vi "VISJS Viewer.vi"(4 "Extra Scripts":string, 5 "FileDependency In":map{path, T1}(c390), 6 "Options":string, 7 "OpenWebBrowser(False)":bool, 8 "error in":errorcluster, 9 "Embedd VISJS Librarya in HTMl File(False)":bool, 10 "HTMLFilePath":path, 11 "LibraryDependency":map{path, T3}(c390)) -> (0 "error out":errorcluster, 3 "HTMLFileContent":string)   [LabVIEW 2020, in "VISJS Viewer.lvlib"] (continued)
{key:\"_setPixelRatio\",value:function(){this.pixelRatio=this._determinePixelRatio()}},{key:\"setTransform\",value:function(){var g=this.getContext();if(void 0===g)throw new Error(\"Could not get canvax context\");g.setTransform(this.pixelRatio,0,0,this.pixelRatio,0,0)}},{key:\"_XconvertDOMtoCanvas\",value:function(g){return(g-this.body.view.translation.x)/this.body.view.scale}},{key:\"_XconvertCanvasToDOM\",value:function(g){return g*this.body.view.scale+this.body.view.translation.x}},{key:\"_YconvertDOMtoCanvas\",value:function(g){return(g-this.body.view.translation.y)/this.body.view.scale}},{key:\"_YconvertCanvasToDOM\",value:function(g){return g*this.body.view.scale+this.body.view.translation.y}},{key:\"canvasToDOM\",value:function(g){return{x:this._XconvertCanvasToDOM(g.x),y:this._YconvertCanvasToDOM(g.y)}}},{key:\"DOMtoCanvas\",value:function(g){return{x:this._XconvertDOMtoCanvas(g.x),y:this._YconvertDOMtoCanvas(g.y)}}}]),g}();var IP=function(){function g(t,A){var e,C,I=this;cn(this,g),this.body=t,this.canvas=A,this.animationSpeed=1/this.renderRefreshRate,this.animationEasingFunction=\"easeInOutQuint\",this.easingTime=0,this.sourceScale=0,this.targetScale=0,this.sourceTranslation=0,this.targetTranslation=0,this.lockedOnNodeId=void 0,this.lockedOnNodeOffset=void 0,this.touchTime=0,this.viewFunction=void 0,this.body.emitter.on(\"fit\",je(e=this.fit).call(e,this)),this.body.emitter.on(\"animationFinished\",(function(){I.body.emitter.emit(\"_stopRendering\")})),this.body.emitter.on(\"unlockNode\",je(C=this.releaseNode).call(C,this))}return kd(g,[{key:\"setOptions\",value:function(){var g=arguments.length>0&&void 0!==arguments[0]?arguments[0]:{};this.options=g}},{key:\"fit\",value:function(g){var t=arguments.length>1&&void 0!==arguments[1]&&arguments[1];g=function(g,t){var A=fe({nodes:t,minZoomLevel:Number.MIN_VALUE,maxZoomLevel:1},null!=g?g:{});if(!Rh(A.nodes))throw new TypeError(\"Nodes has to be an array of ids.\");if(0===A.nodes.length&&(A.nodes=t),!(\"number\"==typeof A.minZoomLevel&&A.minZoomLevel>0))throw new TypeError(\"Min zoom level has to be a number higher than zero.\");if(!(\"number\"==typeof A.maxZoomLevel&&A.minZoomLevel<=A.maxZoomLevel))throw new TypeError(\"Max zoom level has to be a number higher than min zoom level.\");return A}(g,this.body.nodeIndices);var A,e,C=this.canvas.frame.canvas.clientWidth,I=this.canvas.frame.canvas.clientHeight;if(0===C||0===I)e=1,A=XR.getRange(this.body.nodes,g.nodes);else if(!0===t){var i=0;for(var o in this.body.nodes){if(Object.prototype.hasOwnProperty.call(this.body.nodes,o))!0===this.body.nodes[o].predefinedPosition&&(i+=1)}if(i>.5*this.body.nodeIndices.length)return void this.fit(g,!1);A=XR.getRange(this.body.nodes,g.nodes),e=12.662/(this.body.nodeIndices.length+7.4147)+.0964822,e*=Math.min(C/600,I/600)}else{this.body.emitter.emit(\"_resizeNodes\"),A=XR.getRange(this.body.nodes,g.nodes);var n=C/(1.1*Math.abs(A.maxX-A.minX)),r=I/(1.1*Math.abs(A.maxY-A.minY));e=n<=r?n:r}e>g.maxZoomLevel?e=g.maxZoomLevel:e<g.minZoomLevel&&(e=g.minZoomLevel);var s={position:XR.findCenter(A),scale:e,animation:g.animation};this.moveTo(s)}},{key:\"focus\",value:function(g){var t=arguments.length>1&&void 0!==arguments[1]?arguments[1]:{};if(void 0!==this.body.nodes[g]){var A={x:this.body.nodes[g].x,y:this.body.nodes[g].y};t.position=A,t.lockedOnNode=g,this.moveTo(t)}else console.error(\"Node: \"+g+\" cannot be found.\")}},{key:\"moveTo\",value:function(g){if(void 0!==g){if(null!=g.offset){if(null!=g.offset.x){if(g.offset.x=+g.offset.x,!Ym(g.offset.x))throw new TypeError('The option \"offset.x\" has to be a finite number.')}else g.offset.x=0;if(null!=g.offset.y){if(g.offset.y=+g.offset.y,!Ym(g.offset.y))throw new TypeError('The option \"offset.y\" has to be a finite number.')}else g.offset.x=0}else g.offset={x:0,y:0};if(null!=g.position){if(null!=g.position.x){if(g.position.x=+g.position.x,!Ym(g.position.x))throw new TypeError('The option \"position.x\" has to be a finite number.')}else g.position.x=0;if(null!=g.position.y){if(g.position.y=+g.position.y,!Ym(g.position.y))throw new TypeError('The option \"position.y\" has to be a finite number.')}else g.position.x=0}else g.position=this.getViewPosition();if(null!=g.scale){if(g.scale=+g.scale,!(g.scale>0))throw new TypeError('The option \"scale\" has to be a number greater than zero.')}else g.scale=this.body.view.scale;void 0===g.animation&&(g.animation={duration:0}),!1===g.animation&&(g.animation={duration:0}),!0===g.animation&&(g.animation={}),void 0===g.animation.duration&&(g.animation.duration=1e3),void 0===g.animation.easingFunction&&(g.animation.easingFunction=\"easeInOutQuad\"),this.animateView(g)}else g={}}},{key:\"animateView\",value:function(g){if(void 0!==g){this.animationEasingFunction=g.animation.easingFunction,this.releaseNode(),!0===g.locked&&(this.lockedOnNodeId=g.lockedOnNode,this.lockedOnNodeOffset=g.offset),0!=this.easingTime&&this._transitionRedraw(!0),this.sourceScale=this.body.view.scale,this.sourceTranslation=this.body.view.translation,this.targetScale=g.scale,this.body.view.scale=this.targetScale;var t,A,e=this.canvas.DOMtoCanvas({x:.5*this.canvas.frame.canvas.clientWidth,y:.5*this.canvas.frame.canvas.clientHeight}),C=e.x-g.position.x,I=e.y-g.position.y;if(this.targetTranslation={x:this.sourceTranslation.x+C*this.targetScale+g.offset.x,y:this.sourceTranslation.y+I*this.targetScale+g.offset.y},0===g.animation.duration)if(null!=this.lockedOnNodeId)this.viewFunction=je(t=this._lockedRedraw).call(t,this),this.body.emitter.on(\"initRedraw\",this.viewFunction);else this.body.view.scale=this.targetScale,this.body.view.translation=this.targetTranslation,this.body.emitter.emit(\"_requestRedraw\");else this.animationSpeed=1/(60*g.animation.duration*.001)||1/60,this.animationEasingFunction=g.animation.easingFunction,this.viewFunction=je(A=this._transitionRedraw).call(A,this),this.body.emitter.on(\"initRedraw\",this.viewFunction),this.body.emitter.emit(\"_startRendering\")}}},{key:\"_lockedRedraw\",value:function(){var g=this.body.nodes[this.lockedOnNodeId].x,t=this.body.nodes[this.lockedOnNodeId].y,A=this.canvas.DOMtoCanvas({x:.5*this.canvas.frame.canvas.clientWidth,y:.5*this.canvas.frame.canvas.clientHeight}),e=A.x-g,C=A.y-t,I=this.body.view.translation,i={x:I.x+e*this.body.view.scale+this.lockedOnNodeOffset.x,y:I.y+C*this.body.view.scale+this.lockedOnNodeOffset.y};this.body.view.translation=i}},{key:\"releaseNode\",value:function(){void 0!==this.lockedOnNodeId&&void 0!==this.viewFunction&&(this.body.emitter.off(\"initRedraw\",this.viewFunction),this.lockedOnNodeId=void 0,this.lockedOnNodeOffset=void 0)}},{key:\"_transitionRedraw\",value:function(){var g=arguments.length>0&&void 0!==arguments[0]&&arguments[0];this.easingTime+=this.animationSpeed,this.easingTime=!0===g?1:this.easingTime;var t=hv[this.animationEasingFunction](this.easingTime);if(this.body.view.scale=this.sourceScale+(this.targetScale-this.sourceScale)*t,this.body.view.translation={x:this.sourceTranslation.x+(this.targetTranslation.x-this.sourceTranslation.x)*t,y:this.sourceTranslation.y+(this.targetTranslation.y-this.sourceTranslation.y)*t},this.easingTime>=1){var A;if(this.body.emitter.off(\"initRedraw\",this.viewFunction),this.easingTime=0,null!=this.lockedOnNodeId)this.viewFunction=je(A=this._lockedRedraw).call(A,this),this.body.emitter.on(\"initRedraw\",this.viewFunction);this.body.emitter.emit(\"animationFinished\")}}},{key:\"getScale\",value:function(){return this.body.view.scale}},{key:\"getViewPosition\",value:function(){return this.canvas.DOMtoCanvas({x:.5*this.canvas.frame.canvas.clientWidth,y:.5*this.canvas.frame.canvas.clientHeight})}}]),g}();function iP(g){var t,A=g&&g.preventDefault||!1,e=g&&g.container||window,C={},I={keydown:{},keyup:{}},i={};for(t=97;t<=122;t++)i[String.fromCharCode(t)]={code:t-97+65,shift:!1};for(t=65;t<=90;t++)i[String.fromCharCode(t)]={code:t,shift:!0};for(t=0;t<=9;t++)i[\"\"+t]={code:48+t,shift:!1};for(t=1;t<=12;t++)i[\"F\"+t]={code:111+t,shift:!1};for(t=0;t<=9;t++)i[\"num\"+t]={code:96+t,shift:!1};i[\"num*\"]={code:106,shift:!1},i[\"num+\"]={code:107,shift:!1},i[\"num-\"]={code:109,shift:!1},i[\"num/\"]={code:111,shift:!1},i[\"num.\"]={code:110,shift:!1},i.left={code:37,shift:!1},i.up={code:38,shift:!1},i.right={code:39,shift:!1},i.down={code:40,shift:!1},i.space={code:32,shift:!1},i.enter={code:13,shift:!1},i.shift={code:16,shift:void 0},i.esc={code:27,shift:!1},i.backspace={code:8,shift:!1},i.tab={code:9,shift:!1},i.ctrl={code:17,shift:!1},i.alt={code:18,shift:!1},i.delete={code:46,shift:!1},i.pageup={code:33,shift:!1},i.pagedown={code:34,shift:!1},i[\"=\"]={code:187,shift:!1},i[\"-\"]={code:189,shift:!1},i[\"]\"]={code:221,shift:!1},i[\"[\"]={code:219,shift:!1};var o=function(g){r(g,\"keydown\")},n=function(g){r(g,\"keyup\")},r=function(g,t){if(void 0!==I[t][g.keyCode]){for(var e=I[t][g.keyCode],C=0;C<e.length;C++)(void 0===e[C].shift||1==e[C].shift&&1==g.shiftKey||0==e[C].shift&&0==g.shiftKey)&&e[C].fn(g);1==A&&g.preventDefault()}};return C.bind=function(g,t,A){if(void 0===A&&(A=\"keydown\"),void 0===i[g])throw new Error(\"unsupported key: \"+g);void 0===I[A][i[g].code]&&(I[A][i[g].code]=[]),I[A][i[g].code].push({fn:t,shift:i[g].shift})},C.bindAll=function(g,t){for(var A in void 0===t&&(t=\"keydown\"),i)i.hasOwnProperty(A)&&C.bind(A,g,t)},C.getKey=function(g){for(var t in i)if(i.hasOwnProperty(t)){if(1==g.shiftKey&&1==i[t].shift&&g.keyCode==i[t].code)return t;if(0==g.shiftKey&&0==i[t].shift&&g.keyCode==i[t].code)return t;if(g.keyCode==i[t].code&&\"shift\"==t)return t}return\"unknown key, currently not supported\"},C.unbind=function(g,t,A){if(void 0===A&&(A=\"keydown\"),void 0===i[g])throw new Error(\"unsupported key: \"+g);if(void 0!==t){var e=[],C=I[A][i[g].code];if(void 0!==C)for(var o=0;o<C.length;o++)C[o].fn==t&&C[o].shift==i[g].shift||e.push(I[A][i[g].code][o]);I[A][i[g].code]=e}else I[A][i[g].code]=[]},C.reset=function(){I={keydown:{},keyup:{}}},C.destroy=function(){I={keydown:{},keyup:{}},e.removeEventListener(\"keydown\",o,!0),e.removeEventListener(\"keyup\",n,!0)},e.addEventListener(\"keydown\",o,!0),e.addEventListener(\"keyup\",n,!0),C}_e('div.vis-network div.vis-navigation div.vis-button{-webkit-touch-callout:none;background-position:2px 2px;background-repeat:no-repeat;-moz-border-radius:17px;border-radius:17px;cursor:pointer;display:inline-block;height:34px;position:absolute;-webkit-user-select:none;-khtml-user-select:none;-moz-user-select:none;-ms-user-select:none;user-select:none;width:34px}div.vis-network div.vis-navigation div.vis-button:hover{box-shadow:0 0 3px 3px rgba(56,207,21,.3)}div.vis-network div.vis-navigation div.vis-button:active{box-shadow:0 0 1px 3px rgba(56,207,21,.95)}div.vis-network div.vis-navigation div.vis-button.vis-up{background-image:url(\"data:image/png;base64,iVBORw0KGgoAAAANSUhEUgAAAB4AAAAeCAYAAAA7MK6iAAAACXBIWXMAAAsTAAALEwEAmpwYAAAKT2lDQ1BQaG90b3Nob3AgSUNDIHByb2ZpbGUAAHjanVNnVFPpFj333vRCS4iAlEtvUhUIIFJCi4AUkSYqIQkQSoghodkVUcERRUUEG8igiAOOjoCMFVEsDIoK2AfkIaKOg6OIisr74Xuja9a89+bN/rXXPues852zzwfACAyWSDNRNYAMqUIeEeCDx8TG4eQuQIEKJHAAEAizZCFz/SMBAPh+PDwrIsAHvgABeNMLCADATZvAMByH/w/qQplcAYCEAcB0kThLCIAUAEB6jkKmAEBGAYCdmCZTAKAEAGDLY2LjAFAtAGAnf+bTAICd+Jl7AQBblCEVAaCRACATZYhEAGg7AKzPVopFAFgwABRmS8Q5ANgtADBJV2ZIALC3AMDOEAuyAAgMADBRiIUpAAR7AGDIIyN4AISZABRG8lc88SuuEOcqAAB4mbI8uSQ5RYFbCC1xB1dXLh4ozkkXKxQ2YQJhmkAuwnmZGTKBNA/g88wAAKCRFRHgg/P9eM4Ors7ONo62Dl8t6r8G/yJiYuP+5c+rcEAAAOF0ftH+LC+zGoA7BoBt/qIl7gRoXgugdfeLZrIPQLUAoOnaV/Nw+H48PEWhkLnZ2eXk5NhKxEJbYcpXff5nwl/AV/1s+X48/Pf14L7iJIEyXYFHBPjgwsz0TKUcz5IJhGLc5o9H/LcL//wd0yLESWK5WCoU41EScY5EmozzMqUiiUKSKcUl0v9k4t8s+wM+3zUAsGo+AXuRLahdYwP2SycQWHTA4vcAAPK7b8HUKAgDgGiD4c93/+8//UegJQCAZkmScQAAXkQkLlTKsz/HCAAARKCBKrBBG/TBGCzABhzBBdzBC/xgNoRCJMTCQhBCCmSAHHJgKayCQiiGzbAdKmAv1EAdNMBRaIaTcA4uwlW4Dj1wD/phCJ7BKLyBCQRByAgTYSHaiAFiilgjjggXmYX4IcFIBBKLJCDJiBRRIkuRNUgxUopUIFVIHfI9cgI5h1xGupE7yAAygvyGvEcxlIGyUT3UDLVDuag3GoRGogvQZHQxmo8WoJvQcrQaPYw2oefQq2gP2o8+Q8cwwOgYBzPEbDAuxsNCsTgsCZNjy7EirAyrxhqwVqwDu4n1Y8+xdwQSgUXACTYEd0IgYR5BSFhMWE7YSKggHCQ0EdoJNwkDhFHCJyKTqEu0JroR+cQYYjIxh1hILCPWEo8TLxB7iEPENyQSiUMyJ7mQAkmxpFTSEtJG0m5SI+ksqZs0SBojk8naZGuyBzmULCAryIXkneTD5DPkG+Qh8lsKnWJAcaT4U+IoUspqShnlEOU05QZlmDJBVaOaUt2ooVQRNY9aQq2htlKvUYeoEzR1mjnNgxZJS6WtopXTGmgXaPdpr+h0uhHdlR5Ol9BX0svpR+iX6AP0dwwNhhWDx4hnKBmbGAcYZxl3GK+YTKYZ04sZx1QwNzHrmOeZD5lvVVgqtip8FZHKCpVKlSaVGyovVKmqpqreqgtV81XLVI+pXlN9rkZVM1PjqQnUlqtVqp1Q61MbU2epO6iHqmeob1Q/pH5Z/YkGWcNMw09DpFGgsV/jvMYgC2MZs3gsIWsNq4Z1gTXEJrHN2Xx2KruY/R27iz2qqaE5QzNKM1ezUvOUZj8H45hx+Jx0TgnnKKeX836K3hTvKeIpG6Y0TLkxZVxrqpaXllirSKtRq0frvTau7aedpr1Fu1n7gQ5Bx0onXCdHZ4/OBZ3nU9lT3acKpxZNPTr1ri6qa6UbobtEd79up+6Ynr5egJ5Mb6feeb3n+hx9L/1U/W36p/VHDFgGswwkBtsMzhg8xTVxbzwdL8fb8VFDXcNAQ6VhlWGX4YSRudE8o9VGjUYPjGnGXOMk423GbcajJgYmISZLTepN7ppSTbmmKaY7TDtMx83MzaLN1pk1mz0x1zLnm+eb15vft2BaeFostqi2uGVJsuRaplnutrxuhVo5WaVYVVpds0atna0l1rutu6cRp7lOk06rntZnw7Dxtsm2qbcZsOXYBtuutm22fWFnYhdnt8Wuw+6TvZN9un2N/T0HDYfZDqsdWh1+c7RyFDpWOt6azpzuP33F9JbpL2dYzxDP2DPjthPLKcRpnVOb00dnF2e5c4PziIuJS4LLLpc+Lpsbxt3IveRKdPVxXeF60vWdm7Obwu2o26/uNu5p7ofcn8w0nymeWTNz0MPIQ+BR5dE/C5+VMGvfrH5PQ0+BZ7XnIy9jL5FXrdewt6V3qvdh7xc+9j5yn+M+4zw33jLeWV/MN8C3yLfLT8Nvnl+F30N/I/9k/3r/0QCngCUBZwOJgUGBWwL7+Hp8Ib+OPzrbZfay2e1BjKC5QRVBj4KtguXBrSFoyOyQrSH355jOkc5pDoVQfujW0Adh5mGLw34MJ4WHhVeGP45wiFga0TGXNXfR3ENz30T6RJZE3ptnMU85ry1KNSo+qi5qPNo3ujS6P8YuZlnM1VidWElsSxw5LiquNm5svt/87fOH4p3iC+N7F5gvyF1weaHOwvSFpxapLhIsOpZATIhOOJTwQRAqqBaMJfITdyWOCnnCHcJnIi/RNtGI2ENcKh5O8kgqTXqS7JG8NXkkxTOlLOW5hCepkLxMDUzdmzqeFpp2IG0yPTq9MYOSkZBxQqohTZO2Z+pn5mZ2y6xlhbL+xW6Lty8elQfJa7OQrAVZLQq2QqboVFoo1yoHsmdlV2a/zYnKOZarnivN7cyzytuQN5zvn//tEsIS4ZK2pYZLVy0dWOa9rGo5sjxxedsK4xUFK4ZWBqw8uIq2Km3VT6vtV5eufr0mek1rgV7ByoLBtQFr6wtVCuWFfevc1+1dT1gvWd+1YfqGnRs+FYmKrhTbF5cVf9go3HjlG4dvyr+Z3JS0qavEuWTPZtJm6ebeLZ5bDpaql+aXDm4N2dq0Dd9WtO319kXbL5fNKNu7g7ZDuaO/PLi8ZafJzs07P1SkVPRU+lQ27tLdtWHX+G7R7ht7vPY07NXbW7z3/T7JvttVAVVN1WbVZftJ+7P3P66Jqun4lvttXa1ObXHtxwPSA/0HIw6217nU1R3SPVRSj9Yr60cOxx++/p3vdy0NNg1VjZzG4iNwRHnk6fcJ3/ceDTradox7rOEH0x92HWcdL2pCmvKaRptTmvtbYlu6T8w+0dbq3nr8R9sfD5w0PFl5SvNUyWna6YLTk2fyz4ydlZ19fi753GDborZ752PO32oPb++6EHTh0kX/i+c7vDvOXPK4dPKy2+UTV7hXmq86X23qdOo8/pPTT8e7nLuarrlca7nuer21e2b36RueN87d9L158Rb/1tWeOT3dvfN6b/fF9/XfFt1+cif9zsu72Xcn7q28T7xf9EDtQdlD3YfVP1v+3Njv3H9qwHeg89HcR/cGhYPP/pH1jw9DBY+Zj8uGDYbrnjg+OTniP3L96fynQ89kzyaeF/6i/suuFxYvfvjV69fO0ZjRoZfyl5O/bXyl/erA6xmv28bCxh6+yXgzMV70VvvtwXfcdx3vo98PT+R8IH8o/2j5sfVT0Kf7kxmTk/8EA5jz/GMzLdsAAAAgY0hSTQAAeiUAAICDAAD5/wAAgOkAAHUwAADqYAAAOpgAABdvkl/FRgAABphJREFUeNqcV2twU9cR/nbPlVTHxpKRbNnBLyEbPyJisLEcPwgwUMKQtjNJAzNJZkgNNJOmJaZAaDKlxaXDTIBAcJtOOzSYKSkdiimhAdIMjyT4bYgBYxA2BgcUQPLrCiGDR4qt2x+yXTASFt1/957d7zt3z3d39xDCMQWUfgAz/RI/T4pSTAJpAGL8rECAXX7QFQGq9wOHOxYO1oCgjAdJj1wtB095Giv9TFuZAIWHAziATMPhTAwiHgUkYPXFJu92lMP/2MTpB1AKUCVEgNAcleUo1M+2F8TO6crSTncb1QleAOj2OTSX3Ge1p+Va42m5JrnzbnsCE8Ov+EHgpa0LPLvCJjZ/whuIlN8wAcXG+e1LUn9hm238QU84p1Ld83nsXvuO7Lq+LzKYGAT6/dn58m/HJTYf4O3EShkT8Irpzab1Uz9sGevT5+tWn+j6NB4A5hp/5NSr43xjfd5rW5tT9e3OAhCBiCua5/WsDEls/hdvYklZSwDefmrT8eXmtzuDkb5YZ33p9ndylICAVjWxf39xw/5g5Luv/9H84ZWNcwNEypZT87rXjqyJB85UYDMJYN3U7UdLJ6/6JlgqV517teRqf9uTlug8e1zEk27HgD22o98WsTBh8fWxvjm6ApdONbGvse8LM5NUPOm1Cfabuz3nACAgxX0QEFTJAnjNvLJ+Sepb14KRHnN+Ev+1XJOhZs3Qu1mbG97J2NQgsXroa1dtxrGuf8cHi1mUtPTay0lv1DMJSCRVLtoX+FgGgDQNysBAcez89l9nbbsQSji7rlXkEhjPxb/QatHOcFu0M9zz419oFSRhj/3PuaHiyqasv1Con9NGxHAYUsoCxAqImbYSgCWmFbZQwdsur7N0eC4m6tT6/jUZ750Zeb82c+OZGLWh/2p/W+Kfrmy0hIp/aVKpTSIJEqu2QgFx2iE8CwDp0RbH7Ljng/4yXr+XT3QdyhYsodS0slGr0g2OrEUK7eCrKW82SqzCVz3/yfb6vRwM4xn9rN7JkRkOQRLmfJn2LBPxQjDBqp9lD7XbX7X8pKTP160zR2bdeiX5jYeU/nLSTztNkem3XL5eXbltRUkonBxdgZ2IIUmahUxERQSCVT+rK5hzQ89xQ6P8VaaK1f5VmRvqQ4G+lba+nlnlb5brMhvlk7FBiaPzuwQEmEQhg5BOxMjWTncHc2501cQLkjDTsMCWpyuRQxFP0xXIJfp5FyVW4Zy7KajC06ItbiIGg6ZITBxDxIgbrr1jTSM0fibGIHz8O9sKK0GAibEua9spANh4aY2VmcEg+DEkiBgR/L2hYFgGtcErkQQAMVJgBxyy9hboZzv32v+Kpr7qbEECTAIMAoaJa3qPTmNiiAAgJAjk6J5xhu6HDAIgQYGLmI29PocmMcI8MNYvT1ckfzD9H/ub5br4e4Me9WfOKqtyX6Ud2cwC449PRamifDm6Auc0rTXokci+Xo1EAgBckiDuYGLjpTvntcGIA+SFcp6uUAaAI879VhWrRteYAqn/edq758brXJ1327QMhgJcZjA3EBjNrgZjOG1PkAjyTGENMjZPq5ECQ0MDE9ERBqFZrk0OJ3i4x/7vyIjBxGERt3takgVJEAp9xq3f769WiPDNvSsJdT3HDOEASPelmoBRYT3Kzt5uMtwauJEgSOCpwrk1DIJCoNUMwj9v7MweP9XSQ8/hJPp496fZTAICvLqcyv2B7nRbrgCA03JN5h8ub7A8VqpB437xHvsOy3l3cyaB4L2uqxhti1WLMcSgZQCw7+bOooO3Pk4JBZIYYXISMV5sKH59UePM10GESRGpIf/bE92HU452HywSJIGIllctrhp6YAK5+fHds0lLtJFMXNwkV6fFqA29mROefqiMJj1h6um4a5vY/92dKGaBxIhU5zJTWW2cJmEgGOmeb3c8FxAfb9mdf2RzyGGv5MvU7QwuEySwKHFp/c/M71zA/2F7b1RajnYdLAqMukMVu2YcfmDYE2MD7H+7/Xlq6cRIJqm4zXM+qd3TGjVBir43KSLlXjiELe5TsX+3/yW/ST45PaAHbKmccWh12AP93JNZywj0kSABIobpiXRHjtZ6faout2tyZMadGLXBCxBcvl6NfaAz+tKdFmObpzWl2+tIIBACYy0t/yj34M7HvsKUK+CGassvicX7alYDwwq+vykIEqPVa+Q9gdYk5+V+UE7lj3+FGbuBM/X5JUT8QwIVSSSZiTgmoFR2MfiqYFFPfjpkyrfWPopwxP47AP1pK1g9/dqeAAAAAElFTkSuQmCC\");bottom:50px;left:55px}div.vis-network div.vis-navigation div.vis-button.vis-down{background-image:url(\"data:image/png;base64,iVBORw0KGgoAAAANSUhEUgAAAB4AAAAeCAYAAAA7MK6iAAAACXBIWXMAAAsTAAALEwEAmpwYAAAKT2lDQ1BQaG90b3Nob3AgSUNDIHByb2ZpbGUAAHjanVNnVFPpFj333vRCS4iAlEtvUhUIIFJCi4AUkSYqIQkQSoghodkVUcERRUUEG8igiAOOjoCMFVEsDIoK2AfkIaKOg6OIisr74Xuja9a89+bN/rXXPues852zzwfACAyWSDNRNYAMqUIeEeCDx8TG4eQuQIEKJHAAEAizZCFz/SMBAPh+PDwrIsAHvgABeNMLCADATZvAMByH/w/qQplcAYCEAcB0kThLCIAUAEB6jkKmAEBGAYCdmCZTAKAEAGDLY2LjAFAtAGAnf+bTAICd+Jl7AQBblCEVAaCRACATZYhEAGg7AKzPVopFAFgwABRmS8Q5ANgtADBJV2ZIALC3AMDOEAuyAAgMADBRiIUpAAR7AGDIIyN4AISZABRG8lc88SuuEOcqAAB4mbI8uSQ5RYFbCC1xB1dXLh4ozkkXKxQ2YQJhmkAuwnmZGTKBNA/g88wAAKCRFRHgg/P9eM4Ors7ONo62Dl8t6r8G/yJiYuP+5c+rcEAAAOF0ftH+LC+zGoA7BoBt/qIl7gRoXgugdfeLZrIPQLUAoOnaV/Nw+H48PEWhkLnZ2eXk5NhKxEJbYcpXff5nwl/AV/1s+X48/Pf14L7iJIEyXYFHBPjgwsz0TKUcz5IJhGLc5o9H/LcL//wd0yLESWK5WCoU41EScY5EmozzMqUiiUKSKcUl0v9k4t8s+wM+3zUAsGo+AXuRLahdYwP2SycQWHTA4vcAAPK7b8HUKAgDgGiD4c93/+8//UegJQCAZkmScQAAXkQkLlTKsz/HCAAARKCBKrBBG/TBGCzABhzBBdzBC/xgNoRCJMTCQhBCCmSAHHJgKayCQiiGzbAdKmAv1EAdNMBRaIaTcA4uwlW4Dj1wD/phCJ7BKLyBCQRByAgTYSHaiAFiilgjjggXmYX4IcFIBBKLJCDJiBRRIkuRNUgxUopUIFVIHfI9cgI5h1xGupE7yAAygvyGvEcxlIGyUT3UDLVDuag3GoRGogvQZHQxmo8WoJvQcrQaPYw2oefQq2gP2o8+Q8cwwOgYBzPEbDAuxsNCsTgsCZNjy7EirAyrxhqwVqwDu4n1Y8+xdwQSgUXACTYEd0IgYR5BSFhMWE7YSKggHCQ0EdoJNwkDhFHCJyKTqEu0JroR+cQYYjIxh1hILCPWEo8TLxB7iEPENyQSiUMyJ7mQAkmxpFTSEtJG0m5SI+ksqZs0SBojk8naZGuyBzmULCAryIXkneTD5DPkG+Qh8lsKnWJAcaT4U+IoUspqShnlEOU05QZlmDJBVaOaUt2ooVQRNY9aQq2htlKvUYeoEzR1mjnNgxZJS6WtopXTGmgXaPdpr+h0uhHdlR5Ol9BX0svpR+iX6AP0dwwNhhWDx4hnKBmbGAcYZxl3GK+YTKYZ04sZx1QwNzHrmOeZD5lvVVgqtip8FZHKCpVKlSaVGyovVKmqpqreqgtV81XLVI+pXlN9rkZVM1PjqQnUlqtVqp1Q61MbU2epO6iHqmeob1Q/pH5Z/YkGWcNMw09DpFGgsV/jvMYgC2MZs3gsIWsNq4Z1gTXEJrHN2Xx2KruY/R27iz2qqaE5QzNKM1ezUvOUZj8H45hx+Jx0TgnnKKeX836K3hTvKeIpG6Y0TLkxZVxrqpaXllirSKtRq0frvTau7aedpr1Fu1n7gQ5Bx0onXCdHZ4/OBZ3nU9lT3acKpxZNPTr1ri6qa6UbobtEd79up+6Ynr5egJ5Mb6feeb3n+hx9L/1U/W36p/VHDFgGswwkBtsMzhg8xTVxbzwdL8fb8VFDXcNAQ6VhlWGX4YSRudE8o9VGjUYPjGnGXOMk423GbcajJgYmISZLTepN7ppSTbmmKaY7TDtMx83MzaLN1pk1mz0x1zLnm+eb15vft2BaeFostqi2uGVJsuRaplnutrxuhVo5WaVYVVpds0atna0l1rutu6cRp7lOk06rntZnw7Dxtsm2qbcZsOXYBtuutm22fWFnYhdnt8Wuw+6TvZN9un2N/T0HDYfZDqsdWh1+c7RyFDpWOt6azpzuP33F9JbpL2dYzxDP2DPjthPLKcRpnVOb00dnF2e5c4PziIuJS4LLLpc+Lpsbxt3IveRKdPVxXeF60vWdm7Obwu2o26/uNu5p7ofcn8w0nymeWTNz0MPIQ+BR5dE/C5+VMGvfrH5PQ0+BZ7XnIy9jL5FXrdewt6V3qvdh7xc+9j5yn+M+4zw33jLeWV/MN8C3yLfLT8Nvnl+F30N/I/9k/3r/0QCngCUBZwOJgUGBWwL7+Hp8Ib+OPzrbZfay2e1BjKC5QRVBj4KtguXBrSFoyOyQrSH355jOkc5pDoVQfujW0Adh5mGLw34MJ4WHhVeGP45wiFga0TGXNXfR3ENz30T6RJZE3ptnMU85ry1KNSo+qi5qPNo3ujS6P8YuZlnM1VidWElsSxw5LiquNm5svt/87fOH4p3iC+N7F5gvyF1weaHOwvSFpxapLhIsOpZATIhOOJTwQRAqqBaMJfITdyWOCnnCHcJnIi/RNtGI2ENcKh5O8kgqTXqS7JG8NXkkxTOlLOW5hCepkLxMDUzdmzqeFpp2IG0yPTq9MYOSkZBxQqohTZO2Z+pn5mZ2y6xlhbL+xW6Lty8elQfJa7OQrAVZLQq2QqboVFoo1yoHsmdlV2a/zYnKOZarnivN7cyzytuQN5zvn//tEsIS4ZK2pYZLVy0dWOa9rGo5sjxxedsK4xUFK4ZWBqw8uIq2Km3VT6vtV5eufr0mek1rgV7ByoLBtQFr6wtVCuWFfevc1+1dT1gvWd+1YfqGnRs+FYmKrhTbF5cVf9go3HjlG4dvyr+Z3JS0qavEuWTPZtJm6ebeLZ5bDpaql+aXDm4N2dq0Dd9WtO319kXbL5fNKNu7g7ZDuaO/PLi8ZafJzs07P1SkVPRU+lQ27tLdtWHX+G7R7ht7vPY07NXbW7z3/T7JvttVAVVN1WbVZftJ+7P3P66Jqu
